vi "Info.vi"(0 "SystemEvents in":refnum<class "SystemEvents.lvclass">, 1 "event data":T1, 5 "error in (no error)":errorcluster) -> (14 "SystemEvents out":refnum<class "SystemEvents.lvclass">, 19 "error out":errorcluster)   [LabVIEW 2017, in "SystemEvents.lvclass"]
doc: "Fires the Result event with the input parameters in attributes of the event data variant."
uses:
  SystemEvents.lvclass
  SystemEventData/InfoEventData.ctl
  SystemEvents.lvclass/SystemEvents.ctl
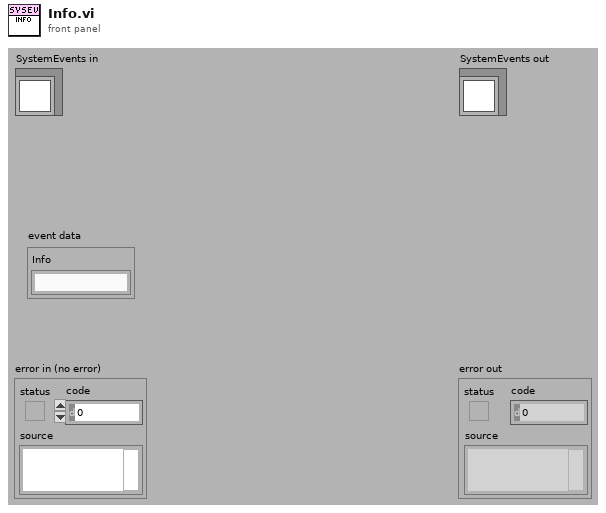
[diagram p1: front panel]
types:
  T1 = typedef "InfoEventData.ctl" = cluster{"Info":string}
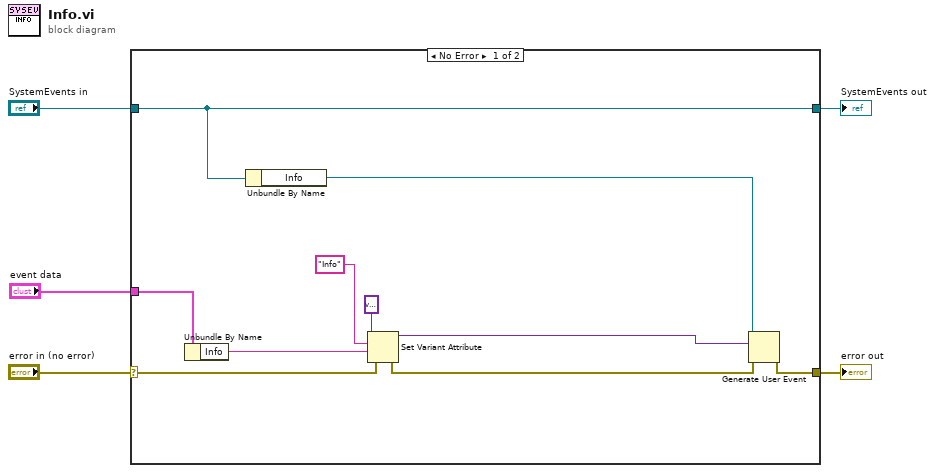
[diagram p0: block diagram]
diagram:
  n1 = case shown="No Error" "error in (no error)" {
    selector: "error in (no error)" -> [w10 w17]
    tunnel: [w14 w17] -> w4
    tunnel: [w15 w16] -> w2
    tunnel: "SystemEvents in" -> [w15 w16]
    tunnel: "event data" -> [w12 _]
    frame No Error {
      n2 = Unbundle By Name(w12) -> ("Info"=w8:string)
      n3 = Unbundle By Name(w15) -> ("Info"=w13:refnum<user-event>)
      n4 = Set Variant Attribute(Variant=variant, name="Info", value=w8, error in=w10) -> (Variant out=w7:variant, error out=w9:errorcluster)  [unwired: 1 out]
      n5 = Generate User Event(user event=w13, event data cluster=w7, error in=w9) -> (error out=w14:errorcluster)  [unwired: 1 in, 1 out]
    }
    frame Error {
    }
  }
  "error out" <- w4
  "SystemEvents out" <- w2
